vi "Msg To Nested.vi"(8 "Alias":string, 9 "Priority?":bool, 10 "Msg":refnum<class "Msg.lvclass">, 11 "Queue Actor in":refnum<class "Queue Actor.lvclass">) -> (0 "error out":errorcluster)   [LabVIEW 2021, in "Queue Actor.lvclass"]
uses:
  Queue Actor.lvclass
  Msg/Msg.lvclass
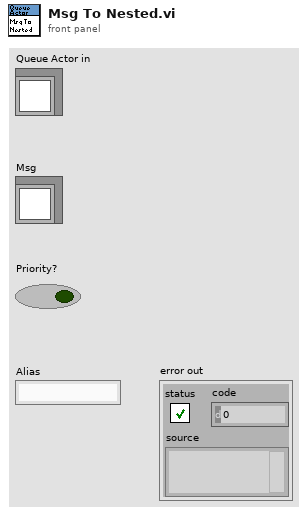
[diagram p1: front panel]
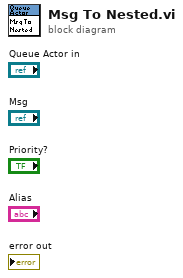
[diagram p0: block diagram]
diagram:
